vi "Crab Drive (Autonomous).vi"(0 "Ignore Turning?":bool, 1 "Execute":bool=TRUE, 2 "Distance (Feet)":dbl=10.0, 3 "Percent Speed":dbl=0.8, 5 "Angle (Degrees)":dbl) -> (4 "Done Executing":bool, 6 "Done":bool, 7 "Traveled":dbl, 8 "Command":dbl)   [LabVIEW 2011]
uses:
  Globals/Encoders Global.vi
  Globals/Autonomous Joystick Emulation.vi
  Auto Drive Emulation.vi
  Globals/Robot Turning.vi
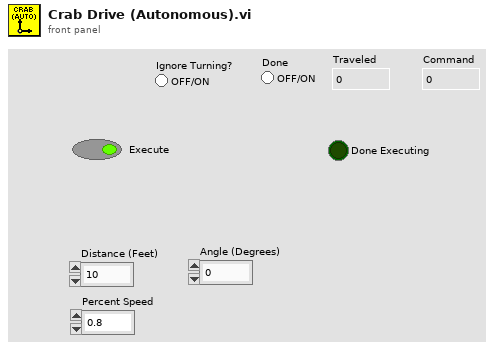
[diagram p1: front panel]
types:
  T1 = typedef "WPI_EncoderDevRef.ctl" = cluster{"DevStatus":errorcluster, "EncoderIndex":T2, "CounterIndex":T3, "DistancePerCount":dbl, "Decoding Type":T4}
  T2 = typedef "FPGA_EncoderIdx.ctl" = enum8{"Enc 0", "Enc 1", "Enc 2", "Enc 3", "Invalid"}
  T3 = typedef "FPGA_CounterCtrSystemIndex.ctl" = enum8{"Ctr 0", "Ctr 1", "Ctr 2", "Ctr 3", "Ctr 4", "Ctr 5", "Ctr 6", "Ctr 7", "Invalid"}
  T4 = typedef "WPI_EncoderType.ctl" = enum16{"1x", "2x", "4x"}
  T5 = cluster{"Front Left":T1, "Front Right":T1, "Rear Left":T1, "Rear Right":T1, "Shooter":T1}
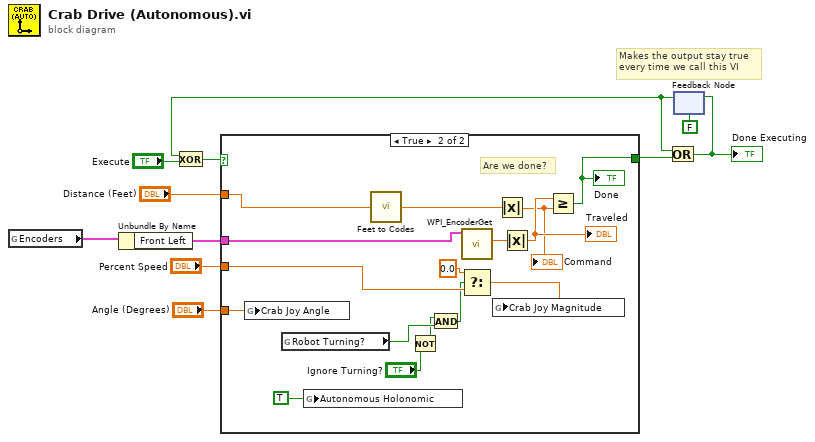
[diagram p0: block diagram]
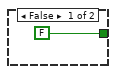
[diagram p2: hidden frame]
diagram:
  # "Makes the output stay true\nevery time we call this VI"
  n1 = global read "Encoders Global.vi" "Encoders"() -> (w5:T5)
  n2 = Unbundle By Name(w5) -> ("Front Left"=w4:T1)
  n3 = feedback #1(FALSE) -> (w2:bool)
  n4 = Exclusive Or(1:"Execute", 2:w2) -> (0:w11:bool)
  n5 = case shown="True" w11 {
    tunnel: [FALSE w28] -> w9
    tunnel: "Percent Speed" -> [_ w16]
    tunnel: "Distance (Feet)" -> [_ w21]
    tunnel: w4 -> [_ w23]
    tunnel: "Angle (Degrees)" -> [_ w20]
    frame False {
    }
    frame True {
      # "Are we done?"
      n6 = global write "Autonomous Joystick Emulation.vi" "Crab Joy Angle"(w20) -> ()
      n7 = global read "Robot Turning.vi" "Robot Turning?"() -> (w19:bool)
      n8 = global write "Auto Drive Emulation.vi" "Autonomous Holonomic"(TRUE ("Autonomous Holonomic")) -> ()
      n9 = call "Feet to Codes.vi"("Feet"=w21) -> ("Codes"=w27:dbl)
      n10 = Not(x="Ignore Turning?") -> (.not. x?=w13:bool)
      n11 = And(x=w13, y=w19) -> (x .and. y?=w15:bool)
      n12 = call <vilib>:"WPI_EncoderGet.vi"("EncoderDevRef"=w23) -> ("Distance"=w26:dbl)  [unwired: 5 in, 5 out]
      n13 = Select(t=0.0, s=w15, f=w16) -> (s? t:f=w17:dbl)
      n14 = global write "Autonomous Joystick Emulation.vi" "Crab Joy Magnitude"(w17) -> ()
      n15 = Absolute Value(x=w27) -> (abs(x)=w24:dbl)
      "Command" <- w24
      n16 = Absolute Value(x=w26) -> (abs(x)=w25:dbl)
      "Traveled" <- w25
      n17 = Greater Or Equal?(x=w25, y=w24) -> (x >= y?=w28:bool)
      "Done" <- w28
    }
  }
  n18 = Or(x=w2, y=w9) -> (x .or. y?=w3:bool)
  "Done Executing" <- w3
  n19 = feedback-in #1(w3) -> ()
